vi "Insert_Into_Array_1D_SubArray.vi"(9 "SubArray IIA":i8[](array[numeric])=[-1, -2], 10 "Index IIA":i32, 11 "Insert into Array 1D":i8[](array[numeric])=[0, 1, 2]) -> (3 "Array 1D IIA":i8[](array[numeric]))   [LabVIEW 2018]
panel:
  out "output array":i8[](array[numeric])
  out "Index":i32
  out "Size":i32
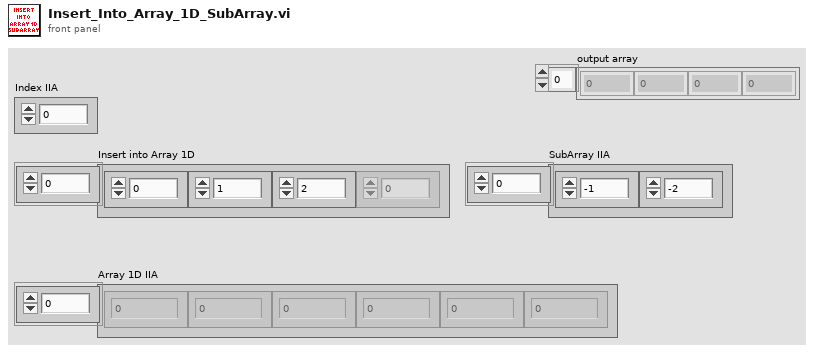
[diagram p1: front panel]
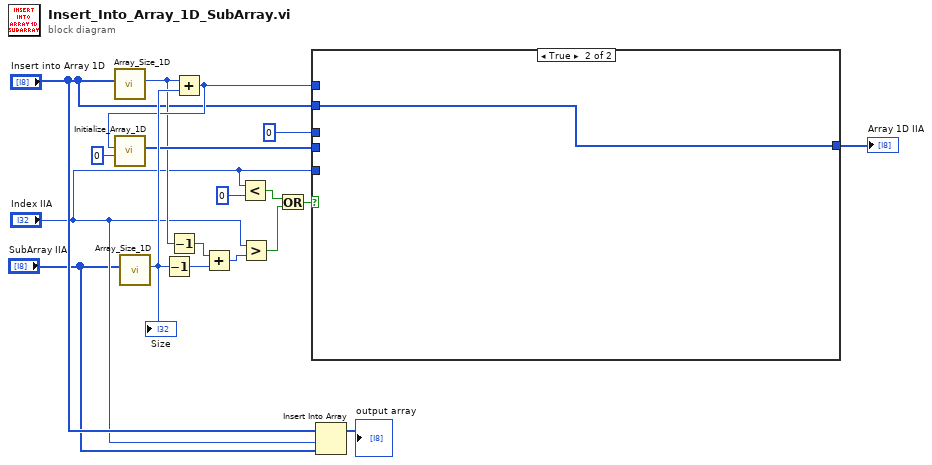
[diagram p0: block diagram]
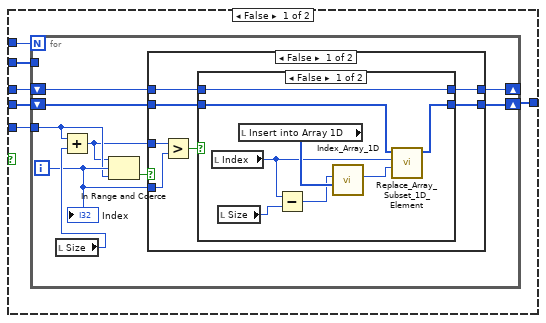
[diagram p2: hidden frame]
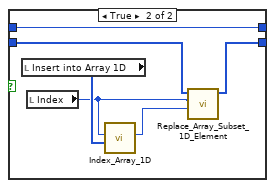
[diagram p3: hidden frame]
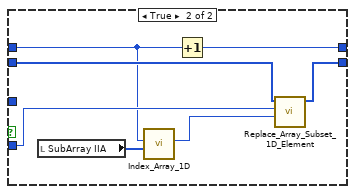
[diagram p4: hidden frame]
diagram:
  n1 = call "Array_Size_1D.vi"("Array"="Insert into Array 1D") -> ("Size"=w9:i32)  [unwired: 10 in]
  n2 = call "Array_Size_1D.vi"("Array"="SubArray IIA") -> ("Size"=w14:i32)  [unwired: 10 in]
  "Size" <- w14
  n3 = Decrement(x=w14) -> (x-1=w17:i32)
  n4 = Decrement(x=w9) -> (x-1=w8:i32)
  n5 = Add(x=w9, y=w14) -> (x+y=w13:i32)
  n6 = call "Initialize_Array_1D.vi"("Value"=i8 0, "Dimension 1D Array"=w13) -> ("Initialized Array 1D"=w12:i8[])  [unwired: 9 in]
  n7 = Add(x=w8, y=w17) -> (x+y=w16:i32)
  n8 = Less?(x="Index IIA", y=0) -> (x < y?=w7:bool)
  n9 = Greater?(x="Index IIA", y=w16) -> (0:w10:bool)
  n10 = Or(x=w7, y=w10) -> (x .or. y?=w15:bool)
  n11 = case shown="True" w15 {
    tunnel: w13 -> [w24 _]
    tunnel: w12 -> [w22 _]
    tunnel: 0 ("Value") -> [w21 _]
    tunnel: "Insert into Array 1D" -> [w23 w62]
    tunnel: "Index IIA" -> [w20 _]
    tunnel: [w19 w62] -> w5
    frame False {
      n12 = for {
        N: w24 -> [_]
        tunnel: w23 -> [_]
        shift-right: [w27] -> _
        shift-left: w21 -> [w28]
        tunnel: w20 -> [w30]
        shift-right: [w25] -> w19
        shift-left: w22 -> [w26]
        i -> [w32]
        n13 = local read "Size"() -> (w33:i32)
        n14 = Add(x=w30, y=w33) -> (x+y=w29:i32)
        n15 = In Range and Coerce(upper limit=w29, x=w32, lower limit=w30) -> (In Range?=w31:bool)  [unwired: 1 out]
        n16 = case shown="False" w31 {
          tunnel: w32 -> [w38 w58]
          tunnel: w29 -> [w39 _]
          tunnel: w28 -> [w37 w56]
          tunnel: [w36 w61] -> w27
          tunnel: w26 -> [w35 w60]
          tunnel: [w34 w59] -> w25
          frame False {
            n17 = Greater?(x=w39, y=w38) -> (0:w40:bool)
            n18 = case shown="False" w40 {
              tunnel: [w41 w54] -> w36
              tunnel: w37 -> [w41 w54]
              tunnel: w35 -> [w43 w51]
              tunnel: [w42 w50] -> w34
              frame False {
                n19 = local read "Index"() -> (w45:i32)
                n20 = local read "Size"() -> (w46:i32)
                n21 = local read "Insert into Array 1D"() -> (w48:i8[])
                n22 = Subtract(x=w45, y=w46) -> (x-y=w47:i32)
                n23 = call "Index_Array_1D.vi"("Index Array 1D"=w48, "Index"=w47) -> ("Value"=w44:i8)  [unwired: 9 in]
                n24 = call "Replace_Array_Subset_1D_Element.vi"("Element RAS"=w44, "Index RAS1D"=w45, "RAS1D"=w43) -> ("New Array RAS1D"=w42:i8[])  [unwired: 8 in]
              }
              frame True {
                n25 = local read "Insert into Array 1D"() -> (w53:i8[])
                n26 = local read "Index"() -> (w52:i32)
                n27 = call "Index_Array_1D.vi"("Index Array 1D"=w53, "Index"=w52) -> ("Value"=w49:i8)  [unwired: 9 in]
                n28 = call "Replace_Array_Subset_1D_Element.vi"("Element RAS"=w49, "Index RAS1D"=w52, "RAS1D"=w51) -> ("New Array RAS1D"=w50:i8[])  [unwired: 8 in]
              }
            }
          }
          frame True {
            n29 = local read "SubArray IIA"() -> (w57:i8[])
            n30 = call "Index_Array_1D.vi"("Index Array 1D"=w57, "Index"=w56) -> ("Value"=w55:i8)  [unwired: 9 in]
            n31 = Increment(x=w56) -> (x+1=w61:i32)
            n32 = call "Replace_Array_Subset_1D_Element.vi"("Element RAS"=w55, "Index RAS1D"=w58, "RAS1D"=w60) -> ("New Array RAS1D"=w59:i8[])  [unwired: 8 in]
          }
        }
        "Index" <- w32
      }
    }
    frame True {
    }
  }
  "Array 1D IIA" <- w5
  n33 = Insert Into Array(array="Insert into Array 1D", index="Index IIA", new element="SubArray IIA") -> (→"output array":i8[])
